vi "test.vi"(8 "error in (no error)":errorcluster, 11 "y":dbl) -> (0 "error out":errorcluster)   [LabVIEW 2019]
panel:
  in  "Boolean":bool
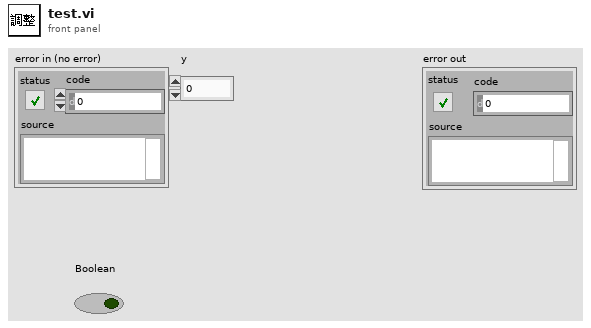
[diagram p1: front panel]
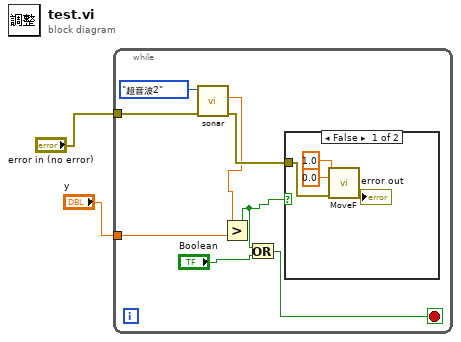
[diagram p0: block diagram]
diagram:
  n1 = while {
    tunnel: "error in (no error)" -> [w7]
    tunnel: "y" -> [w3]
    stop <- w8 stop-if-true
    n2 = call "sonar.vi"("error in (no error)"=w7, "選擇超音波"=enum16{"請選擇超音波", "超音波1", "超音波2", "超音波3", "超音波4"}."超音波2") -> ("error out"=w6:errorcluster, "公分"=w5:dbl)  [unwired: 8 in]
    n3 = Greater?(x=w5, y=w3) -> (0:w4:bool)
    n4 = Or(x=w4, y="Boolean") -> (x .or. y?=w8:bool)
    n5 = case shown="False" w4 {
      tunnel: w6 -> [w11 _]
      frame False {
        n6 = call "MoveF.vi"("X"=1.0, "Y"=0.0, "error in (no error)"=w11) -> ("error out"=→"error out":errorcluster)  [unwired: 12 in]
      }
      frame True {
      }
    }
  }
